vi "Configure Control.vi"(8 "error in (no error)":errorcluster, 10 "control":refnum<vi>, 11 "NT Base in":refnum<class "NT Base.lvclass">) -> (0 "error out":errorcluster, 2 "control out":refnum<vi>, 3 "NT Base out":refnum<class "NT Base.lvclass">)   [LabVIEW 2020, in "PV Access.lvlib" / "PV Data.lvlib" / "NT Base.lvclass"]
doc: "Set the description of <B>control</B> from the value's metadata."
uses:
  NT Base.lvclass
  NT Base.lvclass/NT Base.ctl
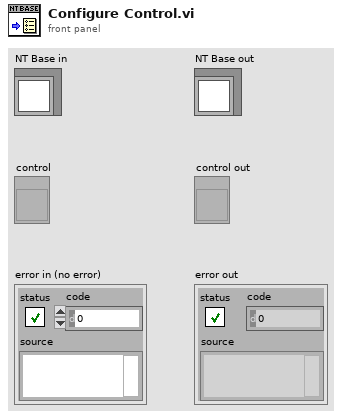
[diagram p1: front panel]
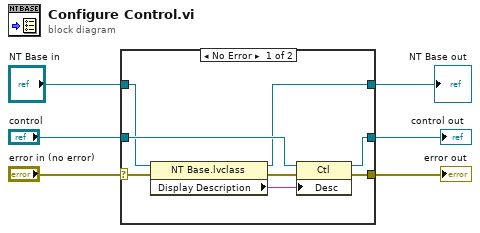
[diagram p0: block diagram]
diagram:
  n1 = case shown="No Error" "error in (no error)" {
    selector: "error in (no error)" -> [w11 w17]
    tunnel: [w13 w17] -> w5
    tunnel: [w9 w16] -> w3
    tunnel: "NT Base in" -> [w10 w16]
    tunnel: "control" -> [w14 w15]
    tunnel: [w7 w15] -> w1
    frame No Error {
      n2 = property class="NT Base.lvclass"(reference=w10, error in=w11) -> (reference out=w9:refnum<class "NT Base.lvclass">, error out=w12:errorcluster, "Display Description"=w8:string)
      n3 = property class="Ctl"(reference=w14, error in=w12, "Desc"=w8) -> (reference out=w7:refnum<vi>, error out=w13:errorcluster)
    }
    frame Error {
    }
  }
  "error out" <- w5
  "NT Base out" <- w3
  "control out" <- w1
